vi "AlliGator Draw Phasor ROIs Overlay.vi"(8 "error in (no error)":errorcluster, 11 "Refnum in":T1) -> (0 "error out":errorcluster, 3 "Refnum out":T1)   [LabVIEW 2021, in "AlliGator Phasor Plot.lvlib"]
doc: "Draws Phasor Plot image ROIs."
uses:
  AlliGator Phasor Plot.lvlib
  <vilib>/vision/Image Controls.llb/IMAQ Image.ctl
  Image/Named ROI Description.ctl
  AlliGator Variables List.ctl
  AlliGator Globals, Variables & Constants.lvlib
  Image/Image.lvlib
  AlliGator ROIs.lvlib
panel:
  # "see the AlliGator License on the block diagram (Ctrl+E or Window:Show Block Diagram)"
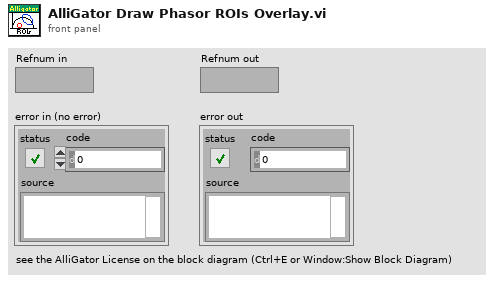
[diagram p1: front panel]
types:
  T1 = typedef "IMAQ Image.ctl" = refnum<image>
  T2 = typedef "Image.lvlib/Named ROI Description.ctl" = cluster{"ROI Descriptor":T3, "ROI Name":string, "Overlay Color":u32}
  T3 = typedef "ROI Descriptor" = cluster{"Global Rectangle":i32[], "Contours":cluster{"ID":enum32{"External", "Internal"}, "Type":u32, "Coordinates":i32[]}[]}
  T4 = typedef "AlliGator Globals, Variables & Constants.lvlib/AlliGator Variables List.ctl" = enum16{"---- GUI ----", "GUI:Initialization Status", "GUI:State Indicators Refnum", "GUI:Original AlliGator Menu Items", "GUI:Current Action Loop State", "GUI:Script in progress", "GUI:Playback", "GUI:Loop Playback", "GUI:Search ROI Used", "GUI:Search ROI", "Decay Graph Max Legend Size", "Intensity Graph Max Legend Size", "Decay Statistics Graph Max Legend Size", "Phasor Graph Max Legend Size", "Phasor Ratio Graph Max Legend Size", "Lifetime Graph Max Legend Size", "---- Files ----", "Files:Export Dataset Frames as Individual Files", "Files:Show Batch Export Help Balloons", "Files:Frames in Dataset", "Files:ptu File Frame Start Indices", "Files:Current Frame in Dataset", "Files:Current Frame Timestamp", "Files:Dataset Loaded", "Files:Dataset Metadata", "Files:Dataset Channel", "Files:Dataset Data Description", "Files:Background Dataset Metadata", "Files:Background Dataset Channel", "Files:Background Dataset Data Description", "Files:Background File Subtraction", "Files:Background File Path", "Files:Background File Pile-up Correction", "Files:Background File Pixel Well Capacity", "Files:Background File Scaling Factor", "Files:Current Dataset Load Settings", "Files:Dataset Path", "Files:ICCD-specific Information", "Files:Macrotime Gate Separation", "------ Python Plugins ------", "Python Plugins:Information", "Python Plugins:Python Session", "Python Plugins:Valid Python Session?", "---- Source Image ----", "Source Image:ROIs", "Source Image:Current ROI", "Source Image:ROI Event Refnum", "X_Source Image Display Range", "X_Source Image Palette Information", "X_Type of Displayed Image", "X_Time Gate Slider", "Source Image:Palette List", "Source Image:Scale", "Source Image:ROI Overlay Color", "Source Image:Overlay to Erase", "Source Image:Is Displayed Image Accumulated", "---- Image Profile Window ----", "Image Profile:Overlay ROI in Source Image", "Image Profile:Window Event Refnum", "Image Profile:IntensityType", "Image Profile:Intensity Average Type", "Image Profile:Intensity-weighted SDV", "Image Profile:Box Profile Type", "Image Profile:Window Open", "Image Profile:Plotted Fit Parameter", "Source Image:White Light Image Modified", "Source Image:Mask Image Modified", "------ Phasor Graph -------", "Phasor Graph:Show Line", "---- Phasor Plot ---", "Phasor Plot:Parameters Changed", "Phasor Plot:FLI Dataset Modified since last Calculation", "Phasor Harmonics Data", "Selected Phasor Harmonics", "Phasor Harmonic Manager Event Refnum", "Phasor Plot:ROIs", "Phasor Plot::Current ROI", "Phasor Plot:ROI Event Refnum", "Phasor Plot:Image Reference Points", "Phasor Plot:Computed", "Phasor Plot:Palette Information", "Phasor Plot:Palette List", "Phasor Ratio Palette Information", "Phasor Ratio Palette List", "Phasor Plot:Image Scale", "Phasor Plot:Image Overlay to Erase", "Phasor Plot:Image Elements to Update", "Current Phasor Plot Calculation Parameters", "Current Phasor Calibration Options", "Phasor Plot:Reset Cumulated Phasor Plot", "Phasor Plot:Reference 1", "Phasor Plot:Lifetime Reference 1", "Phasor Plot:Reference 1 Frequency", "Phasor Plot:Reference 2", "Phasor Plot:Lifetime Reference 2", "Phasor Plot:Reference 2 Frequency", "---- Decay Analysis ----", "Number of Selected Decays to Fit", "LS Fit Results", "LAR Fit Results", "BS Fit Results", "Last Decay Max - Min", "Best Fit Parameters", "Best Fit Parameter Names", "Actual Size X", "Actual Size Y", "Binning X", "Binning Y", "Actual # Gates", "Dataset Number", "Gates to...", "Gates Skipped", "Gates to keep", "Gate Step", "Gate Separation", "Reversed Gates", "Pile-up Correction", "Pixel Well Capacity", "Background Subtracted", "Background Subtraction Method", "Background Definition Range", "Background File (deprecated)", "Number of Dataset Accumulated", "Array of Accumulated Dataset Paths", "Do Averaged Datasets", "Destination File Path", "Process Plot Target", "Use 1/D as Phasor Frequency", "---- Decay Fit Parameter Map -----", "Decay Fit Parameter Map Palette Information", "Decay Fit Parameter Map Palette List", "Local Decay Graph Window Event Refnum", "------- Local Decay Window ---------", "Use normalized IRF for convolution", "----- Miscellaneous ----", "Skippable Dialog Windows Status"}
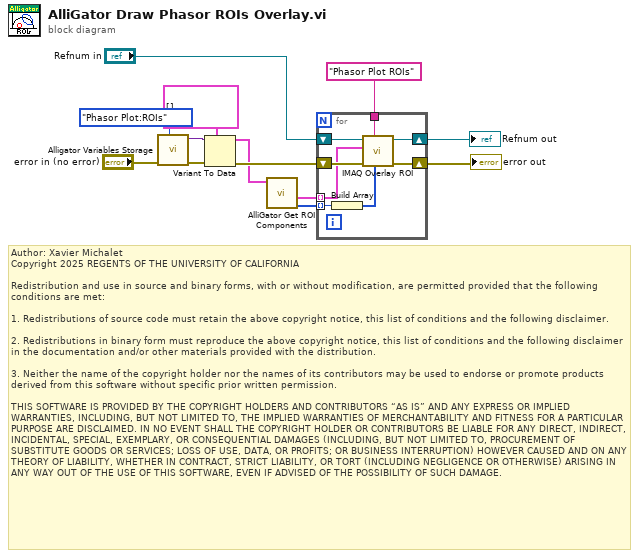
[diagram p0: block diagram]
diagram:
  # "Author: Xavier Michalet\nCopyright 2025 REGENTS OF THE UNIVERSITY OF CALIFORNIA\n\nRedistribution and use in source and binary forms, with or without modification, are permitted provided that the following conditions are met:\n\n1. Redistributions of source code must retain the above copyright notice, this list of conditions and the following disclaimer.\n\n2. Redistributions in binary form must reproduce the above copyright notice, this list of conditions and the following disclaimer in the documentation and/or other materials provided with the distribution.\n\n3. Neither the name of the copyright holder nor the names of its contributors may be used to endorse or promote products derived from this software without specific prior written permission.\n\nTHIS SOFTWARE IS PROVIDED BY THE COPYRIGHT HOLDERS AND CONTRIBUTORS “AS IS” AND ANY EXPRESS OR IMPLIED WARRANTIES, INCLUDING, BUT NOT LIMITED TO, THE IMPLIED WARRANTIES OF MERCHANTABILITY AND FITNESS FOR A PARTICULAR PURPOSE ARE DISCLAIMED. IN NO EVENT SHALL THE COPYRIGHT HOLDER OR CONTRIBUTORS BE LIABLE FOR ANY DIRECT, INDIRECT, INCIDENTAL, SPECIAL, EXEMPLARY, OR CONSEQUENTIAL DAMAGES (INCLUDING, BUT NOT LIMITED TO, PROCUREMENT OF SUBSTITUTE GOODS OR SERVICES; LOSS OF USE, DATA, OR PROFITS; OR BUSINESS INTERRUPTION) HOWEVER CAUSED AND ON ANY THEORY OF LIABILITY, WHETHER IN CONTRACT, STRICT LIABILITY, OR TORT (INCLUDING NEGLIGENCE OR OTHERWISE) ARISING IN ANY WAY OUT OF THE USE OF THIS SOFTWARE, EVEN IF ADVISED OF THE POSSIBILITY OF SUCH DAMAGE."
  n1 = call "Alligator Variables Storage.vi"("AlliGator Variable"=AlliGator_Variables_List."Phasor Plot:ROIs" ("Alligator Variable"), "Error In"="error in (no error)") -> ("Error Out"=w10:errorcluster, "Data out"=w11:variant)  [unwired: 7 in, 1 out]
  n2 = Variant To Data(error in=w10, type=T2[] [] ("ROIs"), Variant=w11) -> (data=w5:T2[], error out=w6:errorcluster)
  n3 = call "AlliGator Get ROI Components.vi"("Stored ROIs"=w5) -> ("Overlay Colors"=w3:u32[], "ROI Descriptors"=w4:T3[])  [unwired: 8 in, 1 out]
  n4 = for {
    tunnel: "Phasor Plot ROIs" ("Group") -> [w21]
    tunnel: w4 -> [w18] mode=indexing
    tunnel: w3 -> [w17] mode=indexing
    shift-right: [w14] -> w2
    shift-left: "Refnum in" -> [w20]
    shift-right: [w15] -> w1
    shift-left: w6 -> [w19]
    n5 = Build Array(w17) -> (w16:u32[])
    n6 = call "IMAQ Overlay ROI"("Colors (Green)"=w16, "Group"=w21, "error in (no error)"=w19, "ROI Descriptor"=w18, "Image"=w20) -> ("error out"=w15:errorcluster, "Image Out"=w14:T1)  [unwired: 5 in]
  }
  "error out" <- w1
  "Refnum out" <- w2
